vi "Get value by Variant.vi"(8 "error in (no error)":errorcluster, 11 "String Column in":refnum<class "String Column.lvclass">) -> (0 "error out":errorcluster, 2 "Variant":variant, 3 "String Column out":refnum<class "String Column.lvclass">)   [LabVIEW 2020, in "Basic Columns.lvlib" / "String Column.lvclass"]
uses:
  String Column.lvclass
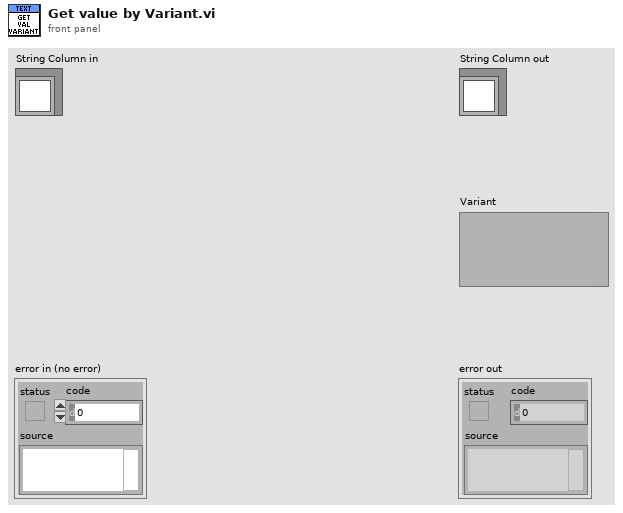
[diagram p1: front panel]
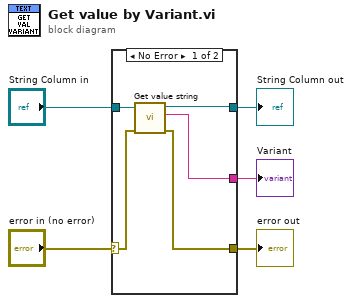
[diagram p0: block diagram]
diagram:
  n1 = case shown="No Error" "error in (no error)" {
    selector: "error in (no error)" -> [w7 w12]
    tunnel: [w6 w12] -> w4
    tunnel: "String Column in" -> [w10 w11]
    tunnel: [w8 w11] -> w2
    tunnel: [w9 _] -> w1
    frame No Error {
      n2 = call-dynamic "Get value string.vi"("error in (no error)"=w7, "Column in"=w10) -> ("error out"=w6:errorcluster, "Value"=w9:string, "Column out"=w8:refnum<class "String Column.lvclass">)  [unwired: 7 in]
    }
    frame Error {
    }
  }
  "error out" <- w4
  "String Column out" <- w2
  "Variant" <- w1
